vi "Data Reshape.vi"() -> ()   [LabVIEW 2020]
uses:
  <vilib>/Utility/miscctls.llb/LVMapReplaceAction.ctl
  <vilib>/Utility/miscctls.llb/LVRowAndColumnTypeDef.ctl
  <vilib>/numeric/Random Number (Range) DBL.vi
panel:
  in  "Classify Type":enum16{"Group By Message", "Group By Time"}(ring)
  out "number of columns":i32
  out "number of rows":i32
  out "Time":dbl
  out "Table":string[][](table)
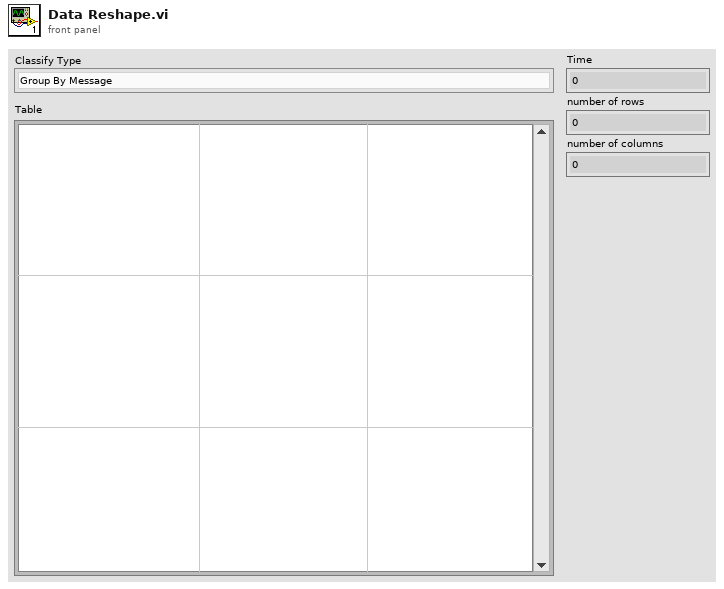
[diagram p1: front panel]
types:
  T1 = typedef "LVMapReplaceAction.ctl" = enum32{"Modify Entry only if found", "Add or Modify Entry", "Delete Entry"}
  T2 = typedef "LVRowAndColumnTypeDef.ctl" = cluster{"Row":i32, "Column":i32}
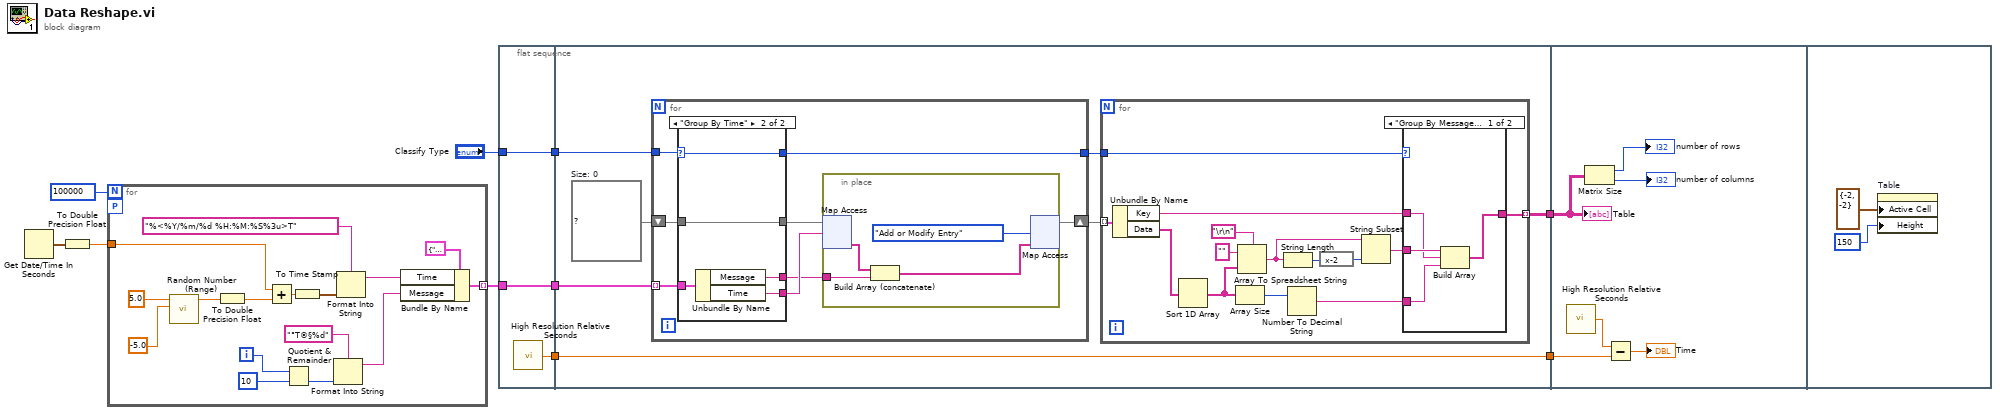
[diagram p0: block diagram]
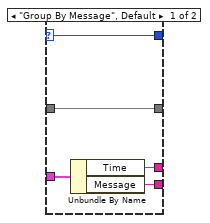
[diagram p2: hidden frame]
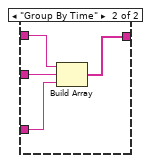
[diagram p3: hidden frame]
diagram:
  n1 = Get Date/Time In Seconds() -> (seconds since 1Jan1904=w10:timestamp)
  n2 = To Double Precision Float(number=w10) -> (double precision float=w9:dbl)
  n3 = for {
    N: 100000 -> [_]
    tunnel: w9 -> [w25]
    tunnel: [w15] -> w7 mode=indexing
    workers-P: _ -> [_]
    i -> [w20]
    n4 = call-poly <vilib>:"Random Number (Range).vi"("lower bound (0)"=-5.0 ("upper bound (100)"), "upper bound (100)"=5.0) -> ("number"=w13:dbl)  [unwired: 9 in]
    n5 = To Double Precision Float(number=w13) -> (double precision float=w24:dbl)
    n6 = Add(x=w25, y=w24) -> (x+y=w23:dbl)
    n7 = Quotient & Remainder(x=w20, y=10) -> (floor(x/y)=w18:i32)  [unwired: 1 out]
    n8 = To Time Stamp(1:w23) -> (0:w22:timestamp)
    n9 = Format Into String(format string="°T®§%d", w18) -> (resulting string=w16:string)  [unwired: 2 in, 1 out]
    n10 = Format Into String(format string="%<%Y/%m/%d %H:%M:%S%3u>T", w22) -> (resulting string=w21:string)  [unwired: 2 in, 1 out]
    n11 = Bundle By Name(cluster=cluster{"Time":string, "Message":string} {"Time"="", "Message"=""} ("Data"), "Time"=w21, "Message"=w16) -> (w15:cluster{"Time":string, "Message":string})
  }
  n12 = flat-sequence {
    tunnel: w7 -> [w29]
    tunnel: [w29] -> w5
    tunnel: [w28] -> w3
    tunnel: "Classify Type" -> [w27]
    tunnel: [w27] -> w1
    tunnel: [w33] -> w6
    tunnel: w5 -> [w35]
    tunnel: [w32] -> w4
    tunnel: w3 -> [w32]
    tunnel: w1 -> [w31]
    tunnel: w6 -> [w83]
    tunnel: w4 -> [w85]
    frame #0 {
      n13 = call <vilib>:"High Resolution Relative Seconds.vi"() -> ("relative seconds"=w28:dbl)
    }
    frame #1 {
      w36 = map{string, string[]} {}  # Size: 0
      n14 = for {
        shift-right: [w41] -> w34
        shift-left: w36 -> [w40]
        tunnel: w35 -> [w44] mode=indexing
        tunnel: w31 -> [w39]
        tunnel: [w38] -> w30
        n15 = case shown="\"Group By Time\"" w39 {
          selector: w39 -> [w46 w54]
          tunnel: w44 -> [w49 w53]
          tunnel: [w48 w50] -> w43
          tunnel: [w47 w51] -> w42
          tunnel: w40 -> [w45 w52]
          tunnel: [w46 w54] -> w38
          tunnel: [w45 w52] -> w37
          frame "Group By Message", Default {
            n16 = Unbundle By Name(w49) -> ("Time"=w47:string, "Message"=w48:string)
          }
          frame "Group By Time" {
            n17 = Unbundle By Name(w53) -> ("Message"=w51:string, "Time"=w50:string)
          }
        }
        n18 = in-place {
          in-place-border: w42 -> [w57]
          n19 = in-place-map #1(w37, w43) -> (w58:string[])  [unwired: 1 in, 1 out]
          n20 = Build Array (concatenate)(w58, w57) -> (w56:string[])
          n21 = in-place-map #1(w56, LVMapReplaceAction."Add or Modify Entry" ("action")) -> (w41:map{string, string[]})  [unwired: 2 out]
        }
      }
      n22 = for {
        tunnel: w34 -> [w72] mode=indexing
        tunnel: [w59] -> w33 mode=indexing
        tunnel: w30 -> [w64]
        n23 = Unbundle By Name(w72) -> ("Key"=w62:string, "Data"=w66:string[])
        n24 = Sort 1D Array(array=w66) -> (sorted array=w65:string[])
        n25 = Array Size(array=w65) -> (size(s)=w63:i32)
        n26 = Array To Spreadsheet String(delimiter (Tab)="\r\n", array=w65, 3:"" ("format string")) -> (spreadsheet string=w69:string)
        n27 = String Length(string=w69) -> (length=w68:i32)
        n28 = Number To Decimal String(number=w63) -> (decimal integer string=w60:string)  [unwired: 1 in]
        n29 = expression code="x-2"(w68) -> (w67:i32)
        n30 = String Subset(string=w69, length (rest)=w67) -> (substring=w61:string)  [unwired: 1 in]
        n31 = case shown="\"Group By Message\", Default" w64 {
          tunnel: w62 -> [w75 w78]
          tunnel: w61 -> [w76 w77]
          tunnel: w60 -> [w74 w80]
          tunnel: [w73 w79] -> w59
          frame "Group By Message", Default {
            n32 = Build Array(w76, w75, w74) -> (w73:string[])
          }
          frame "Group By Time" {
            n33 = Build Array(w78, w77, w80) -> (w79:string[])
          }
        }
      }
    }
    frame #2 {
      n34 = call <vilib>:"High Resolution Relative Seconds.vi"() -> ("relative seconds"=w86:dbl)
      n35 = Matrix Size(0:w83) -> (1:→"number of rows":i32, 2:→"number of columns":i32)
      n36 = Subtract(x=w86, y=w85) -> (x-y=→"Time":dbl)
      "Table" <- w83
    }
    frame #3 {
      n37 = property on="Table" class="Tbl (strict)"("Active Cell"=T2 {"Row"=-2, "Column"=-2} ("Active Cell:Active Cell"), "Height"=u32 150 ("Active Cell:Cell Size:Height")) -> ()  [unwired: 2 in, 2 out]
    }
  }
